vi "Flatten Value.vi"(8 "error in (no error)":errorcluster, 11 "Data Type in":refnum<class "Data Type.lvclass">) -> (0 "error out":errorcluster, 2 "Value":string, 3 "Data Type out":refnum<class "Data Type.lvclass">)   [LabVIEW 2017, in "Data Type.lvclass"]
uses:
  <vilib>/gpm_packages/@cs/data-type-serializer/source/Data Type/Data Type.lvclass
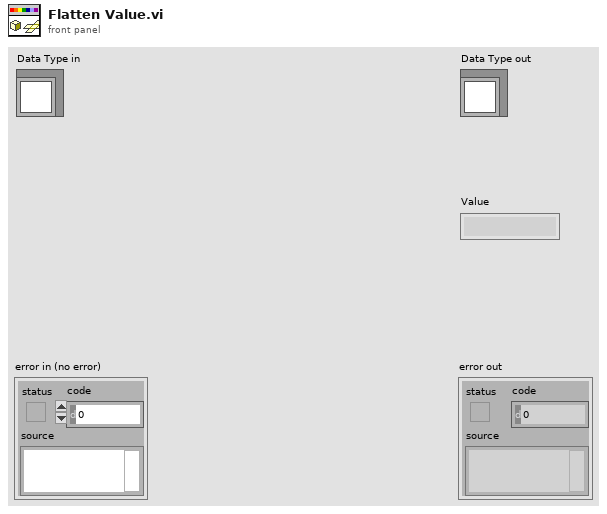
[diagram p1: front panel]
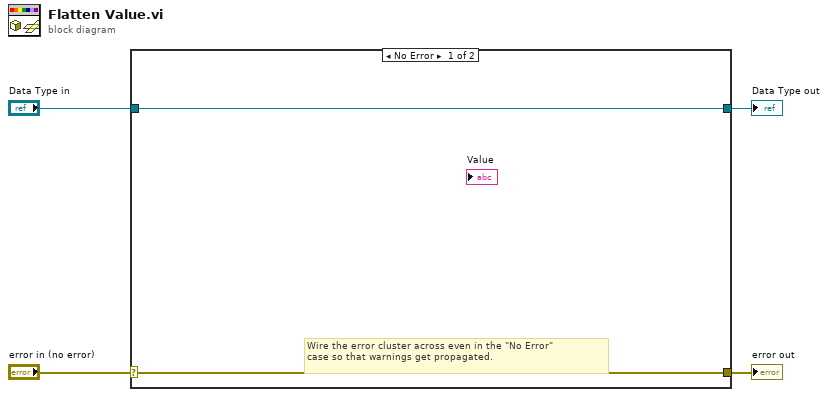
[diagram p0: block diagram]
diagram:
  n1 = case shown="No Error" "error in (no error)" {
    selector: "error in (no error)" -> [w5 w8]
    tunnel: [w5 w8] -> w3
    tunnel: [w6 w7] -> w1
    tunnel: "Data Type in" -> [w6 w7]
    frame No Error {
      # "Wire the error cluster across even in the \"No Error\"\ncase so that warnings get propagated."
    }
    frame Error {
    }
  }
  "error out" <- w3
  "Data Type out" <- w1
